vi "test_SessionsUnreserved_AnyActionOtherThanReserve_ReturnsError.vi"(8 "error in":errorcluster) -> (0 "error out":errorcluster, 2 "result":string, 3 "pass":bool)   [LabVIEW 2020, in "MeasurementServerTests.lvlib" / "Session Reservation Tests.lvlib"]
uses:
  Session Reservation Tests.lvlib
  MeasurementServerTests.lvlib
  Runtime/Measurements/Measurement Plugin Measurement Server/Helpers/Error Strings Global Internal.vi
  da6ffb6f-c1c9-4957-84dd-e9228483c454.vi
  Runtime/APIs/Session Management V1/Session Reservation/Session Reservation.lvclass
  4bbddc2a-be03-47e4-8644-5d4b5205751b.vi
  34973808-273d-4b1e-ac93-8b9a23c2e7c8.vi
  b8e3467f-0abf-4dd6-b6da-3b4f4c560b3c.vi
  44116b28-3318-4200-87c4-820acb1f6e49.vi
  Runtime/Sessions/Instrument Sessions/ISession Factory/ISession Factory.lvclass
  Runtime/APIs/Session Management V1/Session Reservation/Connection.ctl
  Runtime/APIs/Session Management V1/Session Reservation/Connection with Session.ctl
  Runtime/APIs/Session Management V1/Session Reservation/Pin Type.ctl
  Runtime/APIs/Session Management V1/Session Reservation/Initialize and Close Session Behavior.ctl
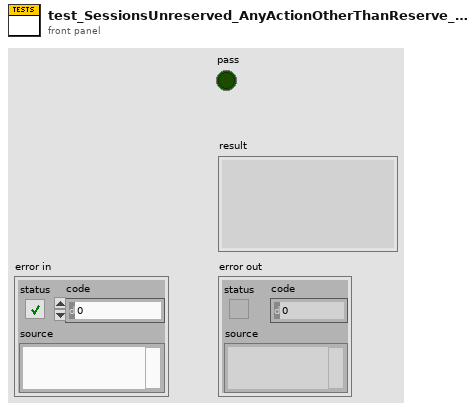
[diagram p1: front panel]
types:
  T1 = typedef "Plug-In SDK Session Management V1.lvlib/Session Reservation.lvclass/Initialize and Close Session Behavior.ctl" = enum16{"Auto", "Initialize and Close", "Attach and Detach", "Initialize and Detach", "Attach and Close"}
  T2 = typedef "Plug-In SDK Session Management V1.lvlib/Session Reservation.lvclass/Pin Type.ctl" = enum16{"DUT and System Pins", "System Pins"}
  T3 = typedef "Plug-In SDK Session Management V1.lvlib/Session Reservation.lvclass/Connection with Session.ctl" = cluster{"connection":T4, "session":variant}
  T4 = typedef "Plug-In SDK Session Management V1.lvlib/Session Reservation.lvclass/Connection.ctl" = cluster{"pin or relay name":string, "site":i32, "instrument type id":string, "channel":string}
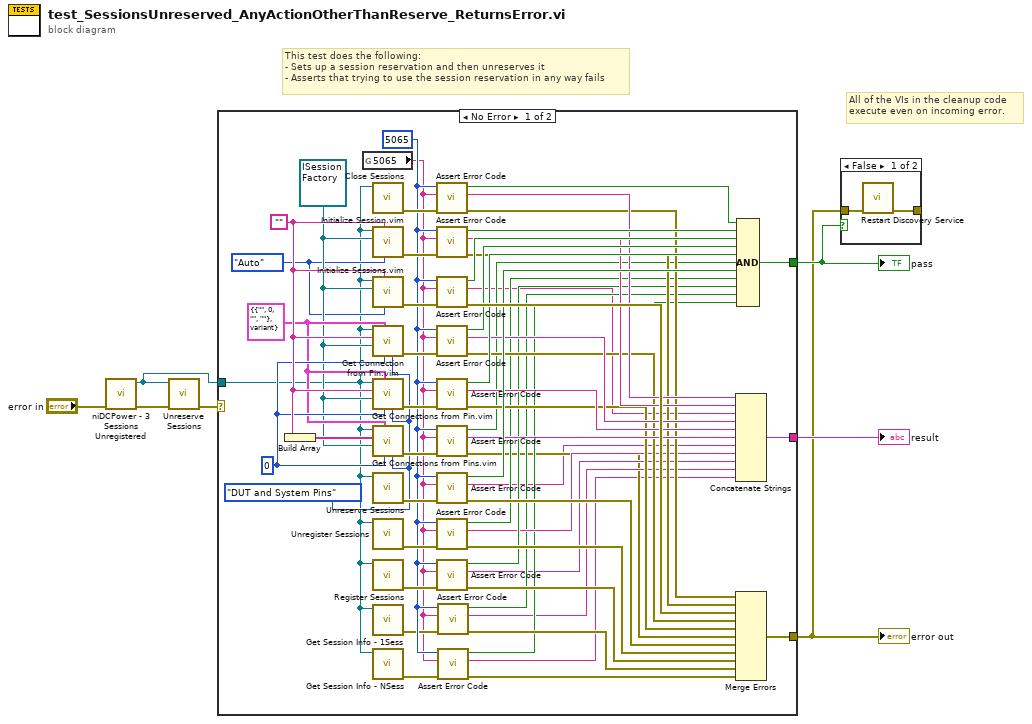
[diagram p0: block diagram]
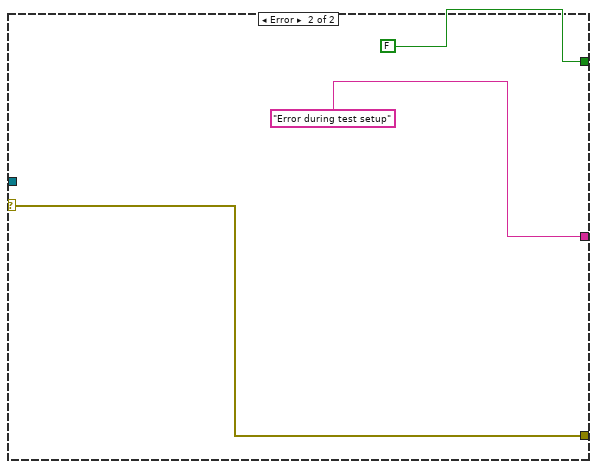
[diagram p2: hidden frame]
diagram:
  # "All of the VIs in the cleanup code\nexecute even on incoming error."
  # "This test does the following:\n- Sets up a session reservation and then unreserves it\n- Asserts that trying to use the session reservation in any way fails"
  n1 = call "niDCPower - 3 Sessions Unregistered.vi"("error in"="error in") -> ("error out"=w2:errorcluster, "session reservation out"=w1:refnum<class "Session Reservation.lvclass">)  [unwired: 9 in]
  n2 = call "Unreserve Sessions.vi"("error in"=w2, "session reservation in"=w1) -> ("error out"=w4:errorcluster)  [unwired: 9 in]
  n3 = case shown="No Error" w4 {
    selector: w4 -> [_ w65]
    tunnel: [w50 w65] -> w5
    tunnel: [w61 FALSE] -> w6
    tunnel: [w56 "Error during test setup" ("f")] -> w7
    tunnel: w1 -> [w24 _]
    frame No Error {
      w25 = Initialize_and_Close_Session_Behavior."Auto" ("initialize and close session behavior")
      w26 = Pin_Type."DUT and System Pins" ("pin type")
      w36 = 0 ("site")
      w38 = ""
      w35 = T3 {"connection"={"pin or relay name"="", "site"=0, "instrument type id"="", "channel"=""}, "session"=variant} ("connection type")
      w34 = refnum<class "ISession Factory.lvclass"> refnum ("instrument")
      w23 = 5065 ("expected error code")
      n4 = Build Array(w38) -> (w37:string[])
      n5 = global read "Error Strings Global Internal.vi" "5065"() -> (w20:string)
      n6 = call "Close Sessions.vi"("session reservation in"=w24) -> ("error out"=w44:errorcluster)  [unwired: 9 in, 1 out]
      n7 = call "Initialize Session.vim"("initialize and close session behavior"=w25, "session type"=w38, "session factory"=w34, "session reservation in"=w24) -> ("error out"=w43:errorcluster)  [unwired: 4 in, 3 out]
      n8 = call "Initialize Sessions.vim"("initialize and close session behavior"=w25, "session type"=w38, "session factory"=w34, "session reservation in"=w24) -> ("error out"=w64:errorcluster)  [unwired: 4 in, 3 out]
      n9 = call "Get Connection from Pin.vim"("pin type"=w26, "site"=w36, "connection type"=w35, "session factory"=w34, "pin or relay name"=w38, "session reservation in"=w24) -> ("error out"=w42:errorcluster)  [unwired: 3 in, 2 out]
      n10 = call "Get Connections from Pin.vim"("pin type"=w26, "site"=w36, "connection type"=w35, "session factory"=w34, "pin or relay name"=w38, "session reservation in"=w24) -> ("error out"=w41:errorcluster)  [unwired: 3 in, 2 out]
      n11 = call "Get Connections from Pins.vim"("pin type"=w26, "site"=w36, "connection type"=w35, "session factory"=w34, "pin or relay names"=w37, "session reservation in"=w24) -> ("error out"=w40:errorcluster)  [unwired: 3 in, 2 out]
      n12 = call "Unreserve Sessions.vi"("session reservation in"=w24) -> ("error out"=w39:errorcluster)  [unwired: 10 in]
      n13 = call "Unregister Sessions.vi"("session reservation in"=w24) -> ("error out"=w33:errorcluster)  [unwired: 9 in, 1 out]
      n14 = call "Register Sessions.vi"("session reservation in"=w24) -> ("error out"=w32:errorcluster)  [unwired: 9 in, 1 out]
      n15 = call "Get Session Info - 1Sess .vi"("session reservation in"=w24) -> ("error out"=w22:errorcluster)  [unwired: 8 in, 2 out]
      n16 = call "Get Session Info - NSess .vi"("session reservation in"=w24) -> ("error out"=w21:errorcluster)  [unwired: 8 in, 2 out]
      n17 = call "Assert Error Code.vi"("error in"=w44, "expected error description"=w20, "expected error code"=w23) -> ("error out"=w49:errorcluster, "details"=w55:string, "error code match?"=w11:bool)  [unwired: 6 in]
      n18 = call "Assert Error Code.vi"("error in"=w43, "expected error description"=w20, "expected error code"=w23) -> ("error out"=w48:errorcluster, "details"=w54:string, "error code match?"=w57:bool)  [unwired: 6 in]
      n19 = call "Assert Error Code.vi"("error in"=w64, "expected error description"=w20, "expected error code"=w23) -> ("error out"=w62:errorcluster, "details"=w8:string, "error code match?"=w63:bool)  [unwired: 6 in]
      n20 = call "Assert Error Code.vi"("error in"=w42, "expected error description"=w20, "expected error code"=w23) -> ("error out"=w47:errorcluster, "details"=w53:string, "error code match?"=w60:bool)  [unwired: 6 in]
      n21 = call "Assert Error Code.vi"("error in"=w41, "expected error description"=w20, "expected error code"=w23) -> ("error out"=w46:errorcluster, "details"=w52:string, "error code match?"=w59:bool)  [unwired: 6 in]
      n22 = call "Assert Error Code.vi"("error in"=w40, "expected error description"=w20, "expected error code"=w23) -> ("error out"=w13:errorcluster, "details"=w51:string, "error code match?"=w12:bool)  [unwired: 6 in]
      n23 = call "Assert Error Code.vi"("error in"=w39, "expected error description"=w20, "expected error code"=w23) -> ("error out"=w45:errorcluster, "details"=w9:string, "error code match?"=w58:bool)  [unwired: 6 in]
      n24 = call "Assert Error Code.vi"("error in"=w33, "expected error description"=w20, "expected error code"=w23) -> ("error out"=w31:errorcluster, "details"=w27:string, "error code match?"=w29:bool)  [unwired: 6 in]
      n25 = call "Assert Error Code.vi"("error in"=w32, "expected error description"=w20, "expected error code"=w23) -> ("error out"=w30:errorcluster, "details"=w14:string, "error code match?"=w28:bool)  [unwired: 6 in]
      n26 = call "Assert Error Code.vi"("error in"=w22, "expected error description"=w20, "expected error code"=w23) -> ("error out"=w19:errorcluster, "details"=w15:string, "error code match?"=w17:bool)  [unwired: 6 in]
      n27 = call "Assert Error Code.vi"("error in"=w21, "expected error description"=w20, "expected error code"=w23) -> ("error out"=w18:errorcluster, "details"=w10:string, "error code match?"=w16:bool)  [unwired: 6 in]
      n28 = Concatenate Strings(w55, w54, w8, w53, w52, w51, w9, w27, w14, w15, w10) -> (w56:string)
      n29 = Merge Errors(w49, w48, w62, w47, w46, w13, w45, w31, w30, w19, w18) -> (w50:errorcluster)
      n30 = Compound Arithmetic op=AND(w11, w57, w63, w60, w59, w12, w58, w29, w28, w17, w16) -> (w61:bool)
    }
    frame Error {
    }
  }
  "error out" <- w5
  "pass" <- w6
  "result" <- w7
  n31 = case shown="False" w6 {
    tunnel: w5 -> [w69 _]
    tunnel: [w68 _] -> _
    frame False {
      n32 = call "Restart Discovery Service.vi"("error in"=w69) -> ("error out"=w68:errorcluster)  [unwired: 10 in]
    }
    frame True {
    }
  }
